vi "CalculatePO2.vi"(8 "A-C open":bool=TRUE, 9 "Gas B pO2":dbl, 10 "Gas A pO2":dbl, 11 "Gases vs time":cluster{"GasA":dbl, "GasB":dbl, "GasC":dbl}(graph)) -> (2 "Estimated pO2":dbl)   [LabVIEW 2013]
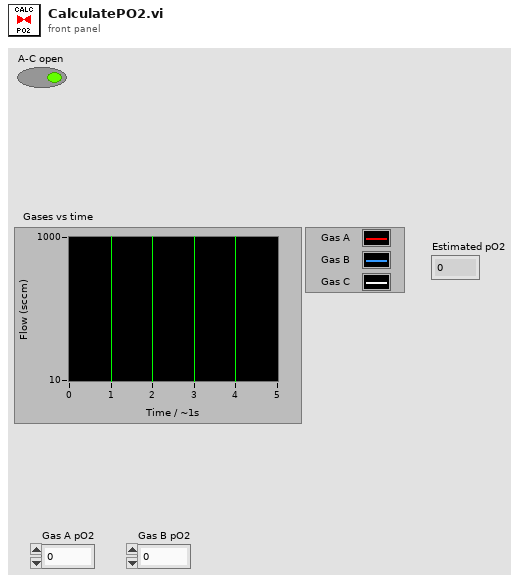
[diagram p1: front panel]
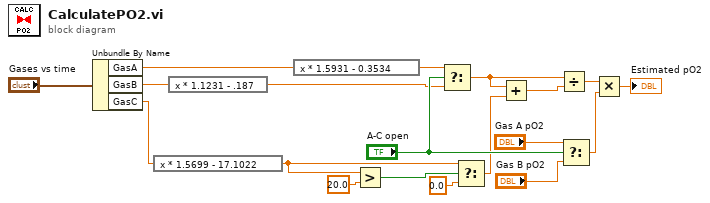
[diagram p0: block diagram]
diagram:
  n1 = Unbundle By Name("Gases vs time") -> ("GasA"=w4:dbl, "GasB"=w5:dbl, "GasC"=w3:dbl)
  n2 = expression code="x * 1.5699 - 17.1022"(w3) -> (w2:dbl)
  n3 = expression code="x * 1.1231 - .187"(w5) -> (w7:dbl)
  n4 = expression code="x * 1.5931 - 0.3534"(w4) -> (w6:dbl)
  n5 = Greater?(x=w2, y=20.0) -> (0:w9:bool)
  n6 = Select(t=w6, s="A-C open", f=w7) -> (s? t:f=w14:dbl)
  n7 = Select(t=w2, s=w9, f=0.0) -> (s? t:f=w1:dbl)
  n8 = Add(x=w14, y=w1) -> (x+y=w15:dbl)
  n9 = Divide(x=w14, y=w15) -> (x/y=w12:dbl)
  n10 = Select(t="Gas A pO2", s="A-C open", f="Gas B pO2") -> (s? t:f=w13:dbl)
  n11 = Multiply(x=w12, y=w13) -> (x*y=→"Estimated pO2":dbl)
